vi "Create.vi"(8 "error in (no error)":errorcluster, 11 "pin map context":T1) -> (0 "error out":errorcluster, 3 "MeasurementContext out":refnum<class "MeasurementContext.lvclass">)   [LabVIEW 2020, in "LoadRegulation.lvlib" / "MeasurementContext.lvclass"]
uses:
  MeasurementContext.lvclass
  RPC Messages/ni_measurementlink_PinMapContext.ctl
  MeasurementContext.lvclass/MeasurementContext.ctl
  LoadRegulation.lvlib
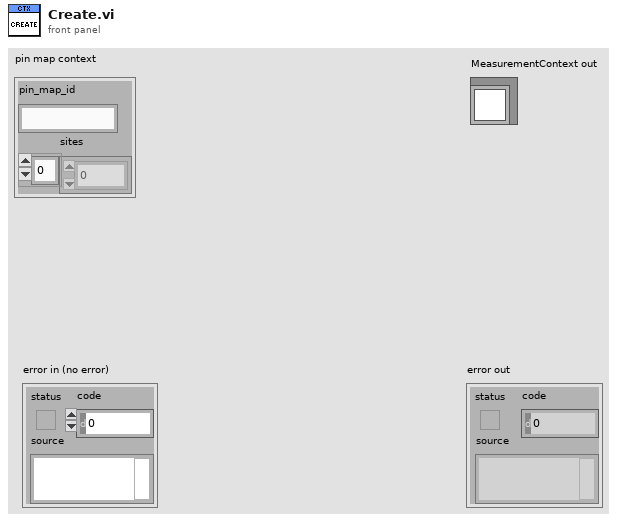
[diagram p1: front panel]
types:
  T1 = typedef "LoadRegulation.lvlib/ni_measurementlink_PinMapContext.ctl" = cluster{"pin_map_id":string, "sites":i32[]}
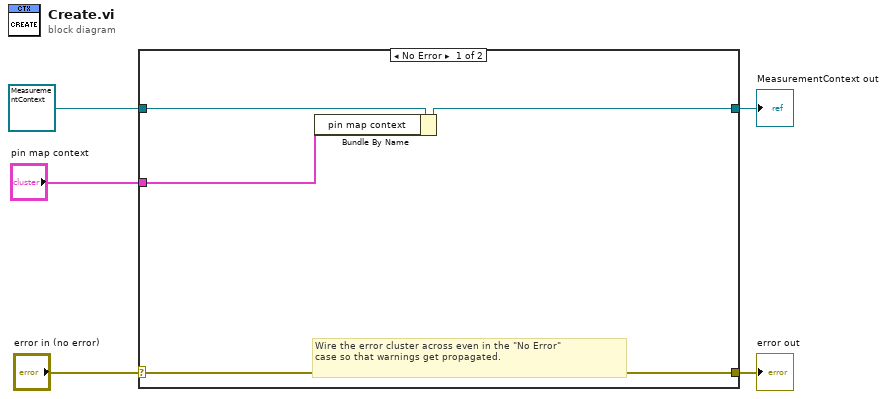
[diagram p0: block diagram]
diagram:
  n1 = case shown="No Error" "error in (no error)" {
    selector: "error in (no error)" -> [w8 w11]
    tunnel: [w8 w11] -> w4
    tunnel: [w7 w10] -> w3
    tunnel: refnum<class "MeasurementContext.lvclass"> refnum ("MeasurementContext.lvclass") -> [w9 w10]
    tunnel: "pin map context" -> [w6 _]
    frame No Error {
      # "Wire the error cluster across even in the \"No Error\"\ncase so that warnings get propagated."
      n2 = Bundle By Name(cluster=w9, "pin map context"=w6) -> (w7:refnum<class "MeasurementContext.lvclass">)
    }
    frame Error {
    }
  }
  "error out" <- w4
  "MeasurementContext out" <- w3
